vi "Delete By Name.vi"(8 "error in (no error)":errorcluster, 10 "Name":string, 11 "LUT in":refnum<class "LUT.lvclass">) -> (0 "error out":errorcluster, 2 "found?":bool, 3 "LUT out":refnum<class "LUT.lvclass">)   [LabVIEW 2017, in "LUT.lvlib" / "LUT.lvclass"]
doc: "Deletes the look up table (LUT) element by name."
uses:
  LUT.lvclass
  LUT.lvclass/LUT.ctl
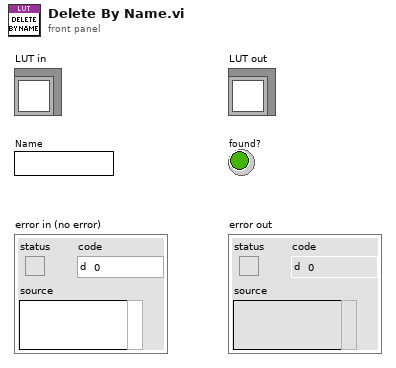
[diagram p1: front panel]
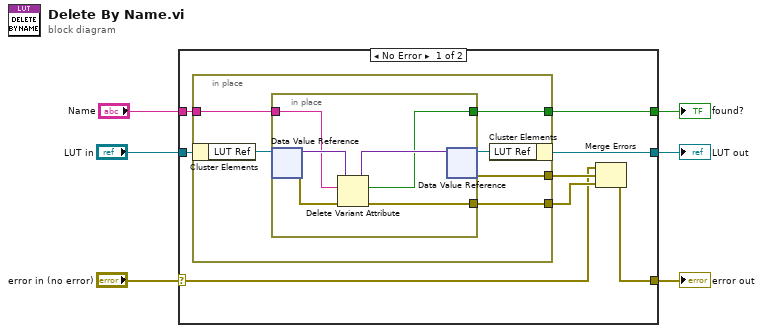
[diagram p0: block diagram]
diagram:
  n1 = case shown="No Error" "error in (no error)" {
    selector: "error in (no error)" -> [w8 w28]
    tunnel: [w7 w28] -> w5
    tunnel: [w13 w27] -> w3
    tunnel: "LUT in" -> [w14 w27]
    tunnel: "Name" -> [w12 _]
    tunnel: [w11 _] -> w1
    frame No Error {
      n2 = in-place {
        in-place-border: w12 -> [w18]
        in-place-border: [w17] -> w11
        in-place-border: [w16] -> w9
        in-place-border: [w15] -> w10
        n3 = in-place-cluster #1(w14) -> ("LUT Ref"=w20:refnum<data-value>)
        n4 = in-place {
          in-place-border: w18 -> [w25]
          in-place-border: [w21] -> w17
          in-place-border: [w23] -> w16
          n5 = in-place-dvr #2(w20) -> (w26:variant, w24:errorcluster)
          n6 = Delete Variant Attribute(4:w24, 6:w25, 7:w26) -> (0:w23:errorcluster, 2:w21:bool, 3:w22:variant)
          n7 = in-place-dvr #2(w22) -> (w19:refnum<data-value>, w15:errorcluster)
        }
        n8 = in-place-cluster #1("LUT Ref"=w19) -> (w13:refnum<class "LUT.lvclass">)
      }
      n9 = Merge Errors(w8, w10, w9) -> (w7:errorcluster)
    }
    frame Error {
    }
  }
  "error out" <- w5
  "LUT out" <- w3
  "found?" <- w1
